vi "PQgetisnull.vi"(7 "error in (no error)":errorcluster, 8 "field_num":i64, 9 "tup_num":i64, 10 "res":u64) -> (0 "error out":errorcluster, 2 "getisnull":u64, 3 "res_out":u64)   [LabVIEW 2019, in "libpqlv64.lvlib"]
doc: "Tests a field for a null value. Row and column numbers start at 0.\nThis function returns 1 if the field is null and 0 if it contains a non-null value. (Note that PQgetvalue will return an empty string, not a null pointer, for a null field."
uses:
  libpqlv64.lvlib
  libpq.dll
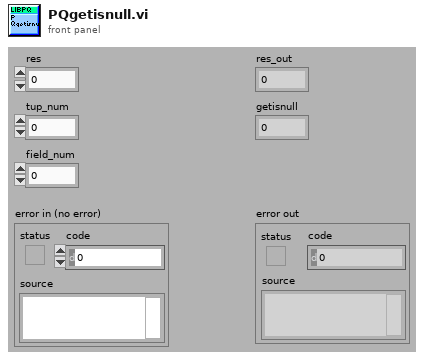
[diagram p1: front panel]
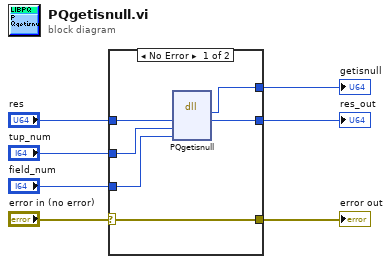
[diagram p0: block diagram]
diagram:
  n1 = case shown="No Error" "error in (no error)" {
    selector: "error in (no error)" -> [w13 w15]
    tunnel: [w13 w15] -> w6
    tunnel: [w12 _] -> w5
    tunnel: "tup_num" -> [w11 _]
    tunnel: "field_num" -> [w10 _]
    tunnel: "res" -> [w9 w14]
    tunnel: [w8 w14] -> w1
    frame No Error {
      n2 = dll-call lib="libpq.*" fn="PQgetisnull"("res"=w9, "tup_num"=w11, "field_num"=w10) -> ("getisnull"=w12:u64, "res"=w8:u64)  [unwired: 5 in, 2 out]
    }
    frame Error {
    }
  }
  "getisnull" <- w5
  "error out" <- w6
  "res_out" <- w1
